vi "Enable.vi"(7 "HomingMode":enum16{"Auto", "Manual"}(ring), 8 "error in (no error)":errorcluster, 11 "Axis in":refnum<class "Axis.lvclass">) -> (0 "error out":errorcluster, 3 "Axis out":refnum<class "Axis.lvclass">)   [LabVIEW 2020, in "Axis.lvclass"]
uses:
  Axis.lvclass
  Axis.lvclass/Axis.ctl
  C:/Users/Jonathan/Documents/Clearpath SDK/CSharp Examples/CLRWrapper/x64/Debug/CLRWrapper.dll
  CSharp Examples/CLRWrapper/x64/Debug/CLRWrapper.dll
  <vilib>/Utility/error.llb/Error Cluster From Error Code.vi
  <vilib>/ErrorRing/Error Ring.xnode
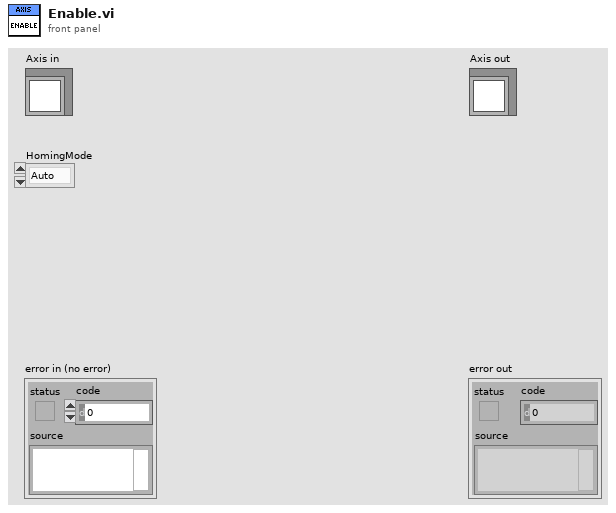
[diagram p1: front panel]
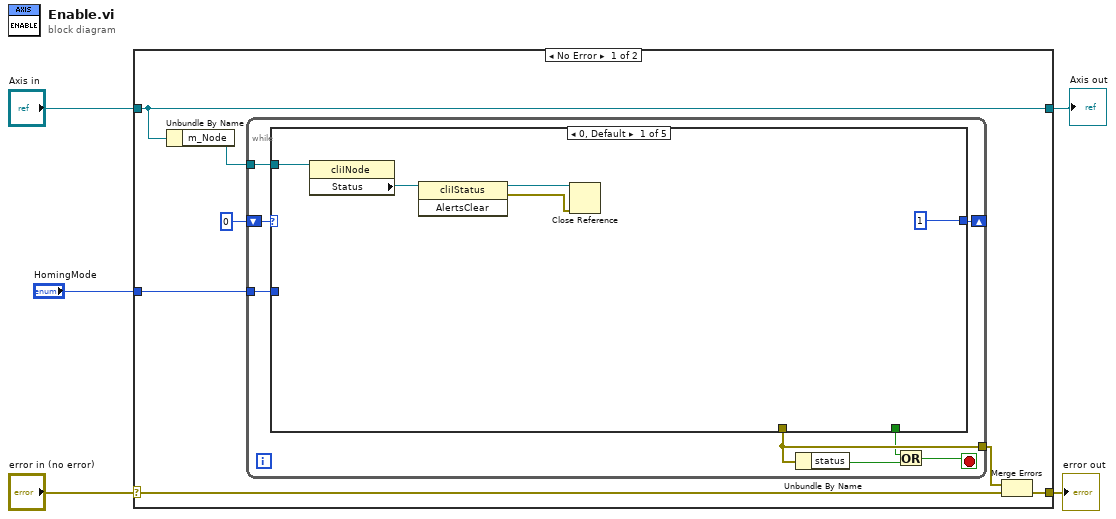
[diagram p0: block diagram]
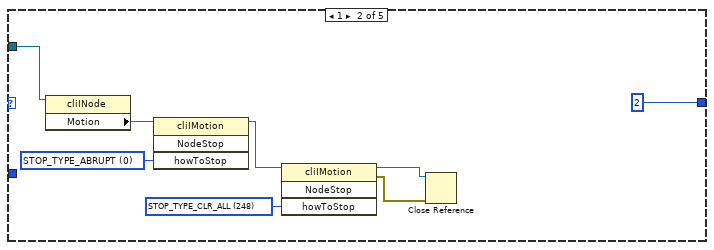
[diagram p2: hidden frame]
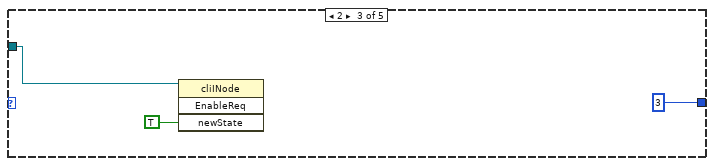
[diagram p3: hidden frame]
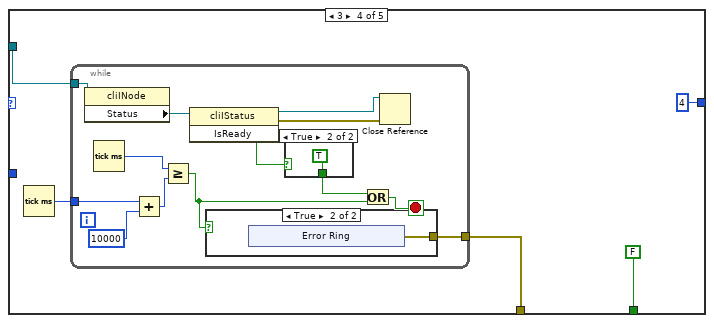
[diagram p4: hidden frame]
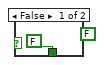
[diagram p6: hidden frame]
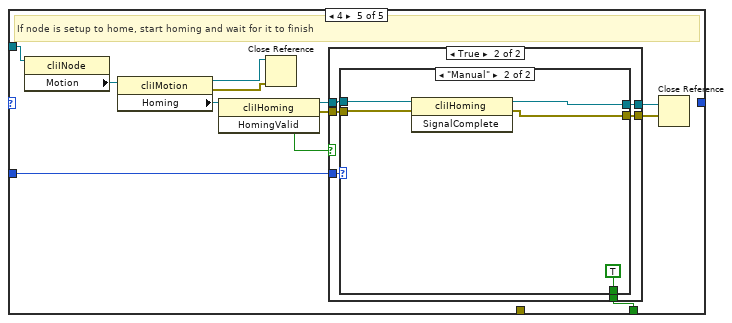
[diagram p7: hidden frame]
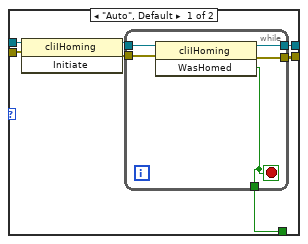
[diagram p9: hidden frame]
diagram:
  n1 = case shown="No Error" "error in (no error)" {
    selector: "error in (no error)" -> [w10 w101]
    tunnel: [w9 w101] -> w4
    tunnel: [w12 w100] -> w2
    tunnel: "Axis in" -> [w12 w100]
    tunnel: "HomingMode" -> [w7 _]
    frame No Error {
      n2 = Unbundle By Name(w12) -> ("m_Node"=w11:refnum<k24>)
      n3 = while {
        tunnel: w11 -> [w20]
        tunnel: [w19] -> w8
        tunnel: w7 -> [w15]
        shift-right: [w14] -> _
        shift-left: 0 -> [w13]
        stop <- w18 stop-if-true
        n4 = case shown="0, Default" w13 {
          tunnel: w20 -> [w25 w29 w35 w41 w71]
          tunnel: [1 2 3 4 _] -> w14
          tunnel: [_ _ _ w39 _] -> w19
          tunnel: [_ _ _ FALSE ("WasHomed") w70] -> w16
          tunnel: w15 -> [_ _ _ _ w63]
          frame 0, Default {
            n5 = property class="cliINode"(reference=w25) -> ("Status"=w24:refnum<k24>)  [unwired: 1 in, 2 out]
            n6 = invoke class="cliIStatus" method="AlertsClear"(reference=w24) -> (reference out=w22:refnum<k24>, error out=w21:errorcluster)  [unwired: 2 in, 1 out]
            n7 = Close Reference(reference=w22, error in (no error)=w21) -> ()  [unwired: 1 out]
          }
          frame 1 {
            w30 = 248 items=["STOP_TYPE_ABRUPT"=0, "STOP_TYPE_RAMP"=1, "STOP_TYPE_IGNORE"=3, "STOP_TYPE_RAMP_AT_DECEL"=4, "STOP_TYPE_ESTOP_ABRUPT"=16, "STOP_TYPE_ESTOP_RAMP"=17, "STOP_TYPE_ESTOP_RAMP_AT_DECEL"=20, "STOP_TYPE_CLR_ESTOP"=24, "STOP_TYPE_CLR_CTRLD"=40, "STOP_TYPE_DISABLE_ABRUPT, STOP_TYPE_DISABLE_RAMP_AT_DECEL, STOP_TYPE_DISABLE_RAMP"=128, "STOP_TYPE_CLR_DISABLE"=136, "STOP_TYPE_ESTOP_DISABLE_RAMP"=145, "STOP_TYPE_CLR_ALL"=248] ("howToStop")
            w32 = 0 items=["STOP_TYPE_ABRUPT"=0, "STOP_TYPE_RAMP"=1, "STOP_TYPE_IGNORE"=3, "STOP_TYPE_RAMP_AT_DECEL"=4, "STOP_TYPE_ESTOP_ABRUPT"=16, "STOP_TYPE_ESTOP_RAMP"=17, "STOP_TYPE_ESTOP_RAMP_AT_DECEL"=20, "STOP_TYPE_CLR_ESTOP"=24, "STOP_TYPE_CLR_CTRLD"=40, "STOP_TYPE_DISABLE_ABRUPT, STOP_TYPE_DISABLE_RAMP_AT_DECEL, STOP_TYPE_DISABLE_RAMP"=128, "STOP_TYPE_CLR_DISABLE"=136, "STOP_TYPE_ESTOP_DISABLE_RAMP"=145, "STOP_TYPE_CLR_ALL"=248] ("howToStop")
            n8 = property class="cliINode"(reference=w29) -> ("Motion"=w33:refnum<k24>)  [unwired: 1 in, 2 out]
            n9 = invoke class="cliIMotion" method="NodeStop"(reference=w33, "howToStop"=w32) -> (reference out=w31:refnum<k24>)  [unwired: 2 in, 3 out]
            n10 = invoke class="cliIMotion" method="NodeStop"(reference=w31, "howToStop"=w30) -> (reference out=w27:refnum<k24>, error out=w26:errorcluster)  [unwired: 2 in, 2 out]
            n11 = Close Reference(reference=w27, error in (no error)=w26) -> ()  [unwired: 1 out]
          }
          frame 2 {
            n12 = invoke class="cliINode" method="EnableReq"(reference=w35, "newState"=TRUE) -> ()  [unwired: 2 in, 4 out]
          }
          frame 3 {
            n13 = Tick Count (ms)() -> (millisecond timer value=w40:u32)
            n14 = while {
              tunnel: w41 -> [w54]
              tunnel: w40 -> [w51]
              tunnel: [w44] -> w39
              stop <- w46 stop-if-true
              n15 = property class="cliINode"(reference=w54) -> ("Status"=w53:refnum<k24>)  [unwired: 1 in, 2 out]
              n16 = Tick Count (ms)() -> (millisecond timer value=w48:u32)
              n17 = Add(x=w51, y=u32 10000) -> (x+y=w49:u32)
              n18 = Greater Or Equal?(x=w48, y=w49) -> (x >= y?=w45:bool)
              n19 = invoke class="cliIStatus" method="IsReady"(reference=w53) -> (reference out=w43:refnum<k24>, error out=w42:errorcluster, "IsReady"=w52:bool)  [unwired: 2 in]
              n20 = case shown="True" w45 {
                tunnel: [_ w55] -> w44
                frame False {
                }
                frame True {
                  n21 = xnode "Error Ring"() -> ("error out"=w55:errorcluster)
                }
              }
              n22 = case shown="True" w52 {
                tunnel: [FALSE TRUE] -> w47
                frame False {
                  (unwired) FALSE
                }
                frame True {
                }
              }
              n23 = Or(x=w47, y=w45) -> (x .or. y?=w46:bool)
              n24 = Close Reference(reference=w43, error in (no error)=w42) -> ()  [unwired: 1 out]
            }
          }
          frame 4 {
            # "If node is setup to home, start homing and wait for it to finish"
            n25 = property class="cliINode"(reference=w71) -> ("Motion"=w74:refnum<k24>)  [unwired: 1 in, 2 out]
            n26 = property class="cliIMotion"(reference=w74) -> (reference out=w69:refnum<k24>, error out=w68:errorcluster, "Homing"=w64:refnum<k24>)  [unwired: 1 in]
            n27 = invoke class="cliIHoming" method="HomingValid"(reference=w64) -> (reference out=w72:refnum<k24>, error out=w67:errorcluster, "HomingValid"=w73:bool)  [unwired: 2 in]
            n28 = Close Reference(reference=w69, error in (no error)=w68) -> ()  [unwired: 1 out]
            n29 = case shown="True" w73 {
              tunnel: w72 -> [w76 w82]
              tunnel: [_ w81] -> w70
              tunnel: [w76 w80] -> w65
              tunnel: [w75 w79] -> w66
              tunnel: w67 -> [w75 w78]
              tunnel: w63 -> [_ w77]
              frame False {
              }
              frame True {
                n30 = case shown="\"Manual\"" w77 {
                  tunnel: w82 -> [w89 w99]
                  tunnel: [w87 TRUE ("WasHomed")] -> w81
                  tunnel: [w83 w96] -> w80
                  tunnel: [w86 w97] -> w79
                  tunnel: w78 -> [w85 w98]
                  frame "Auto", Default {
                    n31 = invoke class="cliIHoming" method="Initiate"(reference=w89, error in=w85) -> (reference out=w88:refnum<k24>, error out=w84:errorcluster)  [unwired: 1 in, 1 out]
                    n32 = while {
                      tunnel: w88 -> [w94]
                      tunnel: [w93] -> w87
                      tunnel: [w92] -> w83
                      tunnel: [w91] -> w86
                      tunnel: w84 -> [w90]
                      stop <- w93 stop-if-true
                      n33 = invoke class="cliIHoming" method="WasHomed"(reference=w94, error in=w90) -> (reference out=w92:refnum<k24>, error out=w91:errorcluster, "WasHomed"=w93:bool)  [unwired: 1 in]
                    }
                  }
                  frame "Manual" {
                    n34 = invoke class="cliIHoming" method="SignalComplete"(reference=w99, error in=w98) -> (reference out=w96:refnum<k24>, error out=w97:errorcluster)  [unwired: 1 in, 1 out]
                  }
                }
              }
            }
            n35 = Close Reference(reference=w65, error in (no error)=w66) -> ()  [unwired: 1 out]
          }
        }
        n36 = Unbundle By Name(w19) -> ("status"=w17:bool)
        n37 = Or(x=w16, y=w17) -> (x .or. y?=w18:bool)
      }
      n38 = Merge Errors(w8, w10) -> (w9:errorcluster)
    }
    frame Error {
    }
  }
  "error out" <- w4
  "Axis out" <- w2
